vi "Receive Challenge Request.vi"(8 "error in (no error)":errorcluster, 11 "Connection in":refnum<class "Connection.lvclass">) -> (0 "error out":errorcluster, 1 "timeout":bool, 2 "Challenge":T1, 3 "Connection out":refnum<class "Connection.lvclass">)   [LabVIEW 2013, in "Connection_GOSPL.lvlib" / "Connection.lvclass"]
uses:
  Connection.lvclass
  challenge request -- cluster.ctl
  Connection.lvclass/Connection.ctl
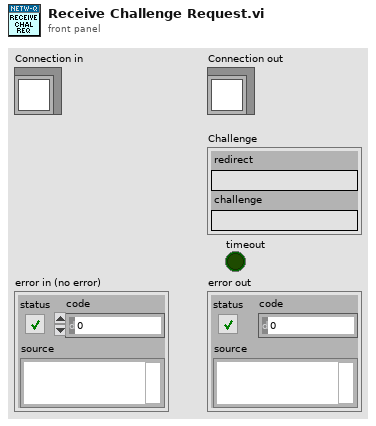
[diagram p1: front panel]
types:
  T1 = typedef "Connection_GOSPL.lvlib/Connection.lvclass/challenge request -- cluster.ctl" = cluster{"redirect":string, "challenge":string}
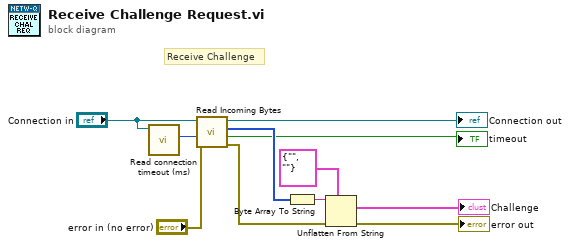
[diagram p0: block diagram]
diagram:
  # "Receive Challenge"
  n1 = call "Read connection timeout (ms).vi"("Connection in"="Connection in") -> ("connection timeout (ms)"=w7:i32)  [unwired: 8 in, 2 out]
  n2 = call-dynamic "Read Incoming Bytes.vi"("error in (no error)"="error in (no error)", "timeout (1000 ms)"=w7, "Connection in"="Connection in") -> ("error out"=w9:errorcluster, "timed out"=→"timeout":bool, "Bytes"=w5:u8[], "Connection out"=→"Connection out":refnum<class "Connection.lvclass">)  [unwired: 4 in, 1 out]
  n3 = Byte Array To String(unsigned byte array=w5) -> (string=w2:string)
  n4 = Unflatten From String(type=T1 {"redirect"="", "challenge"=""} ("Challenge"), binary string=w2, error in (no error)=w9) -> (value=→"Challenge":T1, error out=→"error out":errorcluster)  [unwired: 2 in, 1 out]
